vi "Periodic Tasks.vi"(8 "error in (no error)":errorcluster) -> ()   [LabVIEW 2015]
doc: "This VI runs in parallel to other tasks. It can contain as many user-defined periodic loops as you need. These can carry out PID or other sorts of timed response."
uses:
  <vilib>/Rock Robotics/WPI/Solenoid/WPI_SolenoidValue.ctl
  Robot Global Data.vi
  <vilib>/Rock Robotics/WPI/Solenoid/WPI_SolenoidSetEnum.vi
  <vilib>/Rock Robotics/WPI/Solenoid/Deprecated/WPI_SolenoidSetBool.vi
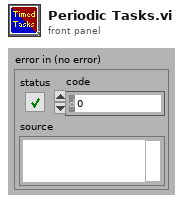
[diagram p1: front panel]
types:
  T1 = typedef "Intake Command.ctl" = cluster{"Closed":bool, "Left Speed":dbl, "Right Speed":dbl}
  T2 = typedef "WPI_SolenoidDevRef.ctl" = cluster{"DevStatus":errorcluster, "Pneumatics Control Module":u8, "Forward Solenoid Channel":T3, "Reverse Solenoid Channel":T3}
  T3 = typedef "WPI_SolenoidChannel.ctl" = enum8{"Solenoid 0", "Solenoid 1", "Solenoid 2", "Solenoid 3", "Solenoid 4", "Solenoid 5", "Solenoid 6", "Solenoid 7", "Invalid"}
  T4 = typedef "WPI_MotorControlDeviceRef.ctl" = cluster{"DeviceStatus":errorcluster, "Type":T5, "PWM":cluster{"PWM Channel":T6, "DeadBand":T7}, "CAN":cluster{"Device Number":u8, "Control Mode":T8, "Semaphore":T9, "Max Vout":dbl, "TalonSRX Control Mode":T10}, "Invert":bool}
  T5 = typedef "WPI_MotorControlType.ctl" = enum16{"PWM", "CAN", "CANTalonSRX"}
  T6 = typedef "FPGA_DIOPWMChannel.ctl" = enum8{"PWM 0", "PWM 1", "PWM 2", "PWM 3", "PWM 4", "PWM 5", "PWM 6", "PWM 7", "PWM 8", "PWM 9", "PWM MXP 0", "PWM MXP 1", "PWM MXP 2", "PWM MXP 3", "PWM MXP 4", "PWM MXP 5", "PWM MXP 6", "PWM MXP 7", "PWM MXP 8", "PWM MXP 9", "Invalid"}
  T7 = typedef "WPI_PWMDeadband.ctl" = cluster{"Name":string, "maxPositivePwm":i32, "minPositivePwm":i32, "centerPwm":i32, "maxNegativePwm":i32, "minNegativePwm":i32, "angularRange":u16}
  T8 = typedef "WPI_CANJaguar_ControlMode.ctl" = enum8{"Percent VBus", "Current", "Speed", "Position", "Voltage"}
  T9 = typedef "Semaphore RefNum" = refnum<k1>
  T10 = typedef "WPI_CANTalonSRX_APIControlMode.ctl" = enum8{"Percent VBus", "Speed", "Position", "Slave", "Unchanged / Invalid", "Voltage Compensation", "Current", "Motion Profile"}
  T11 = typedef "WPI_SolenoidValue.ctl" = enum16{"Off", "On", "Forward", "Reverse"}
  T12 = typedef "Lift Command.ctl" = cluster{"Lift Speed":dbl}
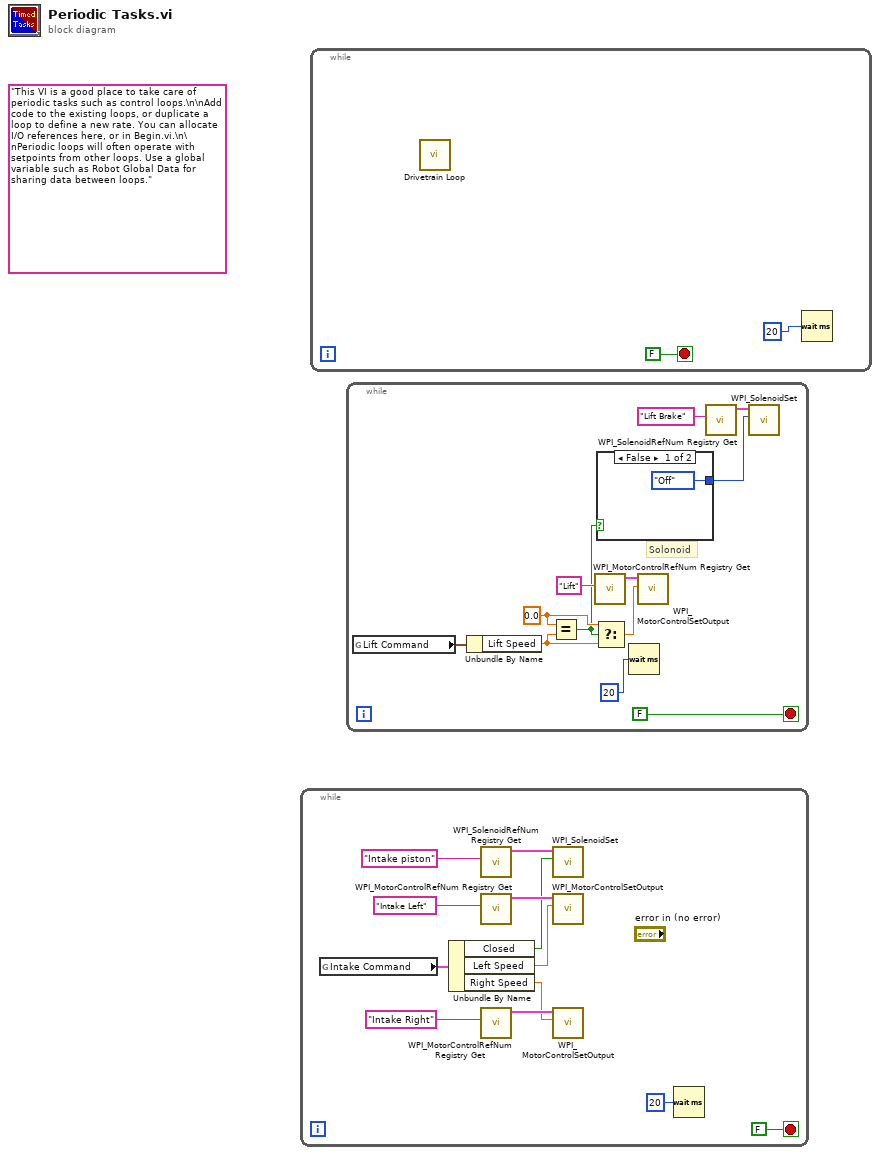
[diagram p0: block diagram]
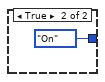
[diagram p2: hidden frame]
diagram:
  (unwired) "This VI is a good place to take care of periodic tasks such as control loops.\n\nAdd code to the existing loops, or duplicate a loop to define a new rate. You can allocate I/O references here, or in Begin.vi.\n\nPeriodic loops will often operate with setpoints from other loops. Use a global variable such as Robot Global Data for sharing data between loops."
  n1 = while {
    stop <- FALSE stop-if-true
    n2 = global read "Robot Global Data.vi" "Intake Command"() -> (w11:T1)
    n3 = Unbundle By Name(w11) -> ("Closed"=w2:bool, "Left Speed"=w6:dbl, "Right Speed"=w4:dbl)
    n4 = call <vilib>:"WPI_SolenoidRefNum Registry Get.vi"("refnum name"="Intake piston") -> ("SolenoidDevRef"=w3:T2)  [unwired: 9 in, 1 out]
    n5 = call <vilib>:"WPI_MotorControlRefNum Registry Get.vi"("refnum name"="Intake Left") -> ("MotorControlDevRef"=w7:T4)  [unwired: 9 in, 1 out]
    n6 = call <vilib>:"WPI_MotorControlRefNum Registry Get.vi"("refnum name"="Intake Right") -> ("MotorControlDevRef"=w5:T4)  [unwired: 9 in, 1 out]
    n7 = call-poly <vilib>:"WPI_SolenoidSet.vi"("Value"=w2, "SolenoidDevRef"=w3) -> ()  [unwired: 8 in, 2 out]
    n8 = call <vilib>:"WPI_MotorControlSetOutput.vi"("Output"=w6, "MotorControlDevRef"=w7) -> ()  [unwired: 7 in, 3 out]
    n9 = call <vilib>:"WPI_MotorControlSetOutput.vi"("Output"=w4, "MotorControlDevRef"=w5) -> ()  [unwired: 7 in, 3 out]
    n10 = Wait (ms)(milliseconds to wait=u32 20) -> ()  [unwired: 1 out]
  }
  n11 = while {
    stop <- FALSE stop-if-true
    n12 = call "Drivetrain Loop.vi"() -> ()  [unwired: 12 in]
    n13 = Wait (ms)(milliseconds to wait=u32 20) -> ()  [unwired: 1 out]
  }
  n14 = while {
    stop <- FALSE stop-if-true
    w24 = 0.0 ("x")
    # "Solonoid"
    n15 = global read "Robot Global Data.vi" "Lift Command"() -> (w18:T12)
    n16 = Unbundle By Name(w18) -> ("Lift Speed"=w17:dbl)
    n17 = Equal?(x=w24, y=w17) -> (x = y?=w21:bool)
    n18 = call <vilib>:"WPI_MotorControlRefNum Registry Get.vi"("refnum name"="Lift") -> ("MotorControlDevRef"=w25:T4)  [unwired: 9 in, 1 out]
    n19 = Select(t=w24, s=w21, f=w17) -> (s? t:f=w19:dbl)
    n20 = case shown="False" w21 {
      tunnel: [WPI_SolenoidValue."Off" ("Value") WPI_SolenoidValue."On" ("Value")] -> w20
      frame False {
      }
      frame True {
      }
    }
    n21 = Wait (ms)(milliseconds to wait=u32 20) -> ()  [unwired: 1 out]
    n22 = call <vilib>:"WPI_MotorControlSetOutput.vi"("Output"=w19, "MotorControlDevRef"=w25) -> ()  [unwired: 7 in, 3 out]
    n23 = call <vilib>:"WPI_SolenoidRefNum Registry Get.vi"("refnum name"="Lift Brake") -> ("SolenoidDevRef"=w22:T2)  [unwired: 9 in, 1 out]
    n24 = call-poly <vilib>:"WPI_SolenoidSet.vi"("Value"=w20, "SolenoidDevRef"=w22) -> ()  [unwired: 8 in, 2 out]
  }
